vi "TextControlledInstrumControlToCommandSingle.vi"(10 "SetGetCommands":string, 11 "Control":refnum<vi>) -> (3 "ControlToCommand":map{refnum<vi>, string[]}(c390))   [LabVIEW 2020]
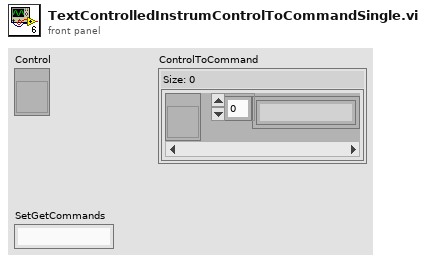
[diagram p1: front panel]
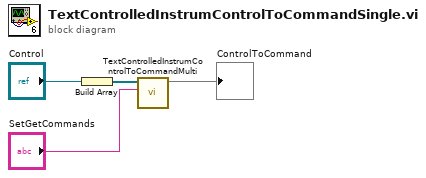
[diagram p0: block diagram]
diagram:
  n1 = Build Array("Control") -> (w3:refnum<vi>[])
  n2 = call "TextControlledInstrumControlToCommandMulti.vi"("SetGetCommands"="SetGetCommands", "Control Array"=w3) -> ("ControlToCommand"=→"ControlToCommand":map{refnum<vi>, string[]})  [unwired: 9 in]
